vi "关键参数解析.vi"(11 "关键参数":u16[](array[numeric])) -> ()   [LabVIEW 2016, in "数据传输系统-03.lvlib"]
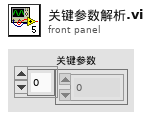
[diagram p1: front panel]
types:
  T1 = cluster{"测量量程":dbl, "测量精度":dbl, "测量间隔":dbl, "消解温度":dbl, "消解时长":dbl, "空白校准时间":timestamp, "曲线截距":dbl, "曲线斜率":dbl, "测量检出限":dbl, "测量信号值":dbl, "线性相关系数":dbl, "二次多项式系数":dbl, "标样校准时间":timestamp, "稀释倍数":dbl, "三项式系数":dbl, "空白标定系数":dbl, "量程系数":dbl, "F0/ORPA":dbl, "F1/ORPB":dbl, "F2/ORPK":dbl, "F3":dbl, "F4":dbl, "F5":dbl, "F6":dbl, "F7":dbl, "X0/滴定数":dbl, "量程":dbl}
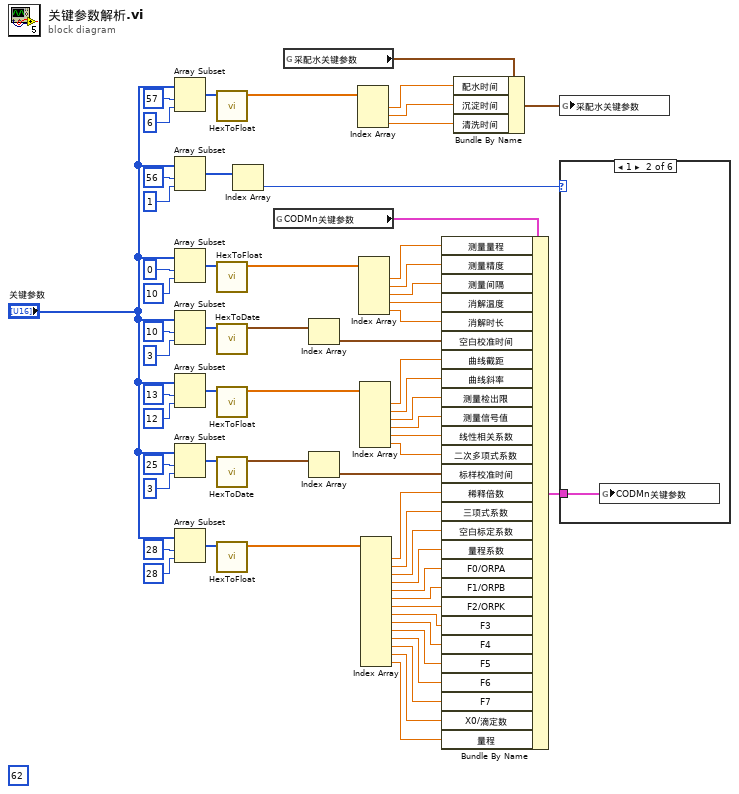
[diagram p0: block diagram]
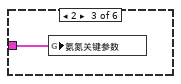
[diagram p3: hidden frame]
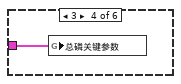
[diagram p4: hidden frame]
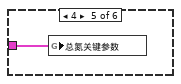
[diagram p5: hidden frame]
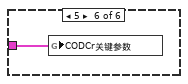
[diagram p6: hidden frame]
diagram:
  (unwired) 62 ("索引")
  n1 = Array Subset(array="关键参数", index=57 ("索引"), length=6 ("长度")) -> (w8:u16[])
  n2 = Array Subset(array="关键参数", index=56 ("索引"), length=1 ("长度")) -> (w11:u16[])
  n3 = Array Subset(array="关键参数", index=0 ("索引"), length=10 ("长度")) -> (w55:u16[])
  n4 = Array Subset(array="关键参数", index=10 ("索引"), length=3 ("长度")) -> (w60:u16[])
  n5 = Array Subset(array="关键参数", index=13 ("索引"), length=12 ("长度")) -> (w44:u16[])
  n6 = Array Subset(array="关键参数", index=25 ("索引"), length=3 ("长度")) -> (w36:u16[])
  n7 = Array Subset(array="关键参数", index=28 ("索引"), length=28 ("长度")) -> (w32:u16[])
  n8 = call "HexToFloat.vi"("数组"=w8) -> ("FLOAT"=w7:sgl[])  [unwired: 10 in]
  n9 = call "HexToFloat.vi"("数组"=w55) -> ("FLOAT"=w54:sgl[])  [unwired: 10 in]
  n10 = call "HexToDate.vi"("数组"=w60) -> ("DATE"=w49:timestamp[])  [unwired: 10 in]
  n11 = call "HexToFloat.vi"("数组"=w44) -> ("FLOAT"=w43:sgl[])  [unwired: 10 in]
  n12 = call "HexToDate.vi"("数组"=w36) -> ("DATE"=w35:timestamp[])  [unwired: 10 in]
  n13 = call "HexToFloat.vi"("数组"=w32) -> ("FLOAT"=w33:sgl[])  [unwired: 10 in]
  n14 = Index Array(array=w11) -> (element=w12:u16)  [unwired: 1 in]
  n15 = global read "全局1.vi" "CODMn关键参数"() -> (w63:T1)
  n16 = global read "全局1.vi" "采配水关键参数"() -> (w6:cluster{"配水时间":dbl, "沉淀时间":dbl, "清洗时间":dbl})
  n17 = Index Array(array=w49) -> (element=w48:timestamp)  [unwired: 1 in]
  n18 = Index Array(array=w35) -> (element=w34:timestamp)  [unwired: 1 in]
  n19 = Index Array(array=w7) -> (element #1=w5:sgl, element #2=w4:sgl, element #3=w3:sgl)  [unwired: 3 in]
  n20 = Index Array(array=w54) -> (element #1=w53:sgl, element #2=w52:sgl, element #3=w51:sgl, element #4=w50:sgl, element #5=w47:sgl)  [unwired: 5 in]
  n21 = Index Array(array=w43) -> (element #1=w42:sgl, element #2=w41:sgl, element #3=w40:sgl, element #4=w39:sgl, element #5=w38:sgl, element #6=w37:sgl)  [unwired: 6 in]
  n22 = Index Array(array=w33) -> (element #1=w29:sgl, element #2=w28:sgl, element #3=w27:sgl, element #4=w26:sgl, element #5=w25:sgl, element #6=w24:sgl, element #7=w23:sgl, element #8=w22:sgl, element #9=w21:sgl, element #10=w20:sgl, element #11=w19:sgl, element #12=w18:sgl, element #13=w17:sgl, element #14=w16:sgl)  [unwired: 14 in]
  n23 = Bundle By Name(cluster=w63, "测量量程"=w53, "测量精度"=w52, "测量间隔"=w51, "消解温度"=w50, "消解时长"=w47, "空白校准时间"=w48, "曲线截距"=w42, "曲线斜率"=w41, "测量检出限"=w40, "测量信号值"=w39, "线性相关系数"=w38, "二次多项式系数"=w37, "标样校准时间"=w34, "稀释倍数"=w29, "三项式系数"=w28, "空白标定系数"=w27, "量程系数"=w26, "F0/ORPA"=w25, "F1/ORPB"=w24, "F2/ORPK"=w23, "F3"=w22, "F4"=w21, "F5"=w20, "F6"=w19, "F7"=w18, "X0/滴定数"=w17, "量程"=w16) -> (w62:T1)
  n24 = Bundle By Name(cluster=w6, "配水时间"=w5, "沉淀时间"=w4, "清洗时间"=w3) -> (w2:cluster{"配水时间":dbl, "沉淀时间":dbl, "清洗时间":dbl})
  n25 = global write "全局1.vi" "采配水关键参数"(w2) -> ()
  n26 = case shown="1" w12 {
    tunnel: w62 -> [_ w64 w65 w66 w67 w68]
    frame 0, Default {
    }
    frame 1 {
      n27 = global write "全局1.vi" "CODMn关键参数"(w64) -> ()
    }
    frame 2 {
      n28 = global write "全局1.vi" "氨氮关键参数"(w65) -> ()
    }
    frame 3 {
      n29 = global write "全局1.vi" "总磷关键参数"(w66) -> ()
    }
    frame 4 {
      n30 = global write "全局1.vi" "总氮关键参数"(w67) -> ()
    }
    frame 5 {
      n31 = global write "全局1.vi" "CODCr关键参数"(w68) -> ()
    }
  }
